vi "DIM_DIO.update bit.vi"(0 "i ref in":refnum<vi>, 1 "badValue":bool, 2 "bitValue":bool, 3 "ms timeout (10000)":i32=10000, 5 "error in (no error)":errorcluster, 6 "bitQuality":i32) -> (14 "i ref out":refnum<vi>, 17 "timed out":bool, 19 "error out":errorcluster)   [LabVIEW 2014, in "DIM_DIO.lvlib"]
doc: "Takes the bit and updates the attribute data and the DIM service."
uses:
  DIM_DIO.lvlib
  CS_Core/CSApplicationBaseClasses/DigiIOBase/DigiIOBase.directionType.ctl
  CS_Core/CSApplicationBaseClasses/DigiIOBase/DigiIOBase.serviceType.ctl
  CS_Core/CSApplicationBaseClasses/DigiIOBase/DigiIOBase.lvlib
  CS_Core/CSSystem/CoreLib/CoreLib.lvlib
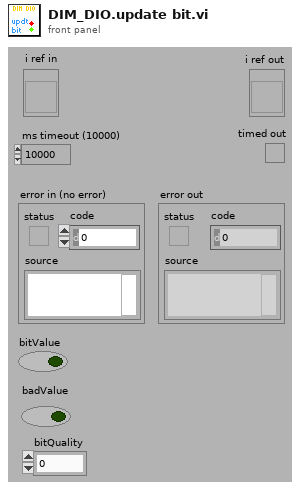
[diagram p1: front panel]
types:
  T1 = typedef "DigiIOBase.lvlib/DigiIOBase.serviceType.ctl" = enum16{"bit", "word"}
  T2 = typedef "DigiIOBase.lvlib/DigiIOBase.directionType.ctl" = enum16{"unknown", "update actual value", "update nominal value", "update both"}
  T3 = typedef "UtilityLib.lvlib/UtilityLib.valueStatus.ctl" = enum16{"no info available", "stand by/off", "on", "warning", "alarm/malfunction", "not implemented", "user action required", "important information", "system default", "control default", "indicator default", "button default"}
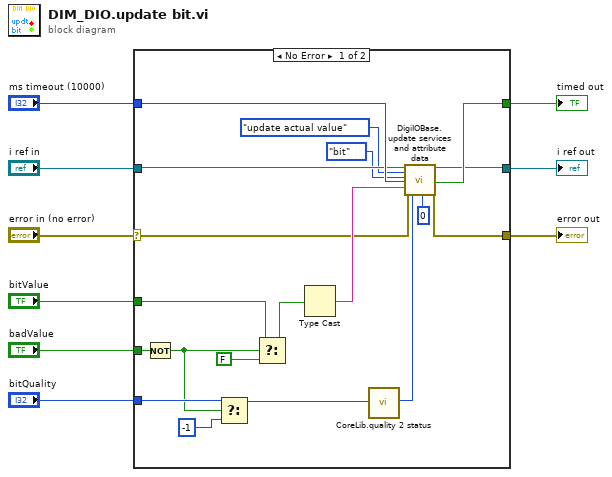
[diagram p0: block diagram]
diagram:
  n1 = case shown="No Error" "error in (no error)" {
    selector: "error in (no error)" -> [w11 w29]
    tunnel: "i ref in" -> [w23 w30]
    tunnel: "bitValue" -> [w18 _]
    tunnel: "ms timeout (10000)" -> [w25 _]
    tunnel: [w22 w30] -> w6
    tunnel: [w10 w29] -> w5
    tunnel: "badValue" -> [w28 _]
    tunnel: "bitQuality" -> [w27 _]
    tunnel: [w24 _] -> w1
    frame No Error {
      n2 = Not(x=w28) -> (.not. x?=w19:bool)
      n3 = Select(t=w27, s=w19, f=-1) -> (s? t:f=w14:i32)
      n4 = Select(t=w18, s=w19, f=FALSE) -> (s? t:f=w16:bool)
      n5 = Type Cast(x=w16) -> (*(type *) &x=w15:string)  [unwired: 1 in]
      n6 = call "CoreLib.quality 2 status.vi"("quality"=w14) -> ("valueStatus"=w13:T3)  [unwired: 18 in]
      n7 = call "DigiIOBase.update services and attribute data.vi"("i ref in"=w23, "direction"=DigiIOBase.directionType."update actual value", "service"=DigiIOBase.serviceType."bit", "ms timeout (10000)"=w25, "value"=w15, "error in (no error)"=w11, "quality"=w13, "index"=0) -> ("i ref out"=w22:refnum<vi>, "timed out"=w24:bool, "error out"=w10:errorcluster)  [unwired: 9 in]
    }
    frame Error {
    }
  }
  "error out" <- w5
  "i ref out" <- w6
  "timed out" <- w1
